vi "UpdateClibWithNewB.vi"(8 "error in (no error)":errorcluster, 11 "MagSpec_Bella in":refnum<class "MagSpec_Bella.lvclass">) -> (0 "error out":errorcluster, 3 "MagSpec_Bella out":refnum<class "MagSpec_Bella.lvclass">)   [LabVIEW 2013, in "MagSpec_Bella.lvclass"]
uses:
  MagSpec_Bella.lvclass
  MagSpec_Bella.lvclass/MagSpec_Bella.ctl
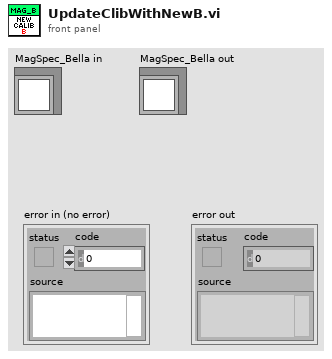
[diagram p1: front panel]
types:
  T1 = typedef "Calibration_Pixel_based.ctl" = cluster{"y1(pixel)":dbl[], "y2(pixel)":dbl[], "dp/B [MeV/C/B] (pixel)":dbl[], "energyDependence Input(pixel)":dbl[], "bending angle [deg](pixel)":dbl[], "total path(pixel)":dbl[], "pixel angle (y)(pixel)":dbl[], "energy dependence (pixel)":dbl[], "charge compensation (pixel)":dbl[], "Momentum [MeV/C](pixel)":dbl[], "angular compensation(pixel)":dbl[]}
  T2 = typedef "CameraSettings_File.ctl" = cluster{"FOV [mm]":dbl, "Left edge [mm]":dbl, "ROI Y offset":dbl, "ROI height":dbl, "ROI X offset":dbl, "ROI width":dbl, "Y center pixel":dbl, "Y Start":dbl, "Y End":dbl, "X Start":dbl, "X End":dbl, "rot [deg]":dbl}
  T3 = typedef "2D.ctl" = cluster{"dp":dbl[][], "chargeCompensation":dbl[][], "angle":dbl[][], "Momentum":dbl[][]}
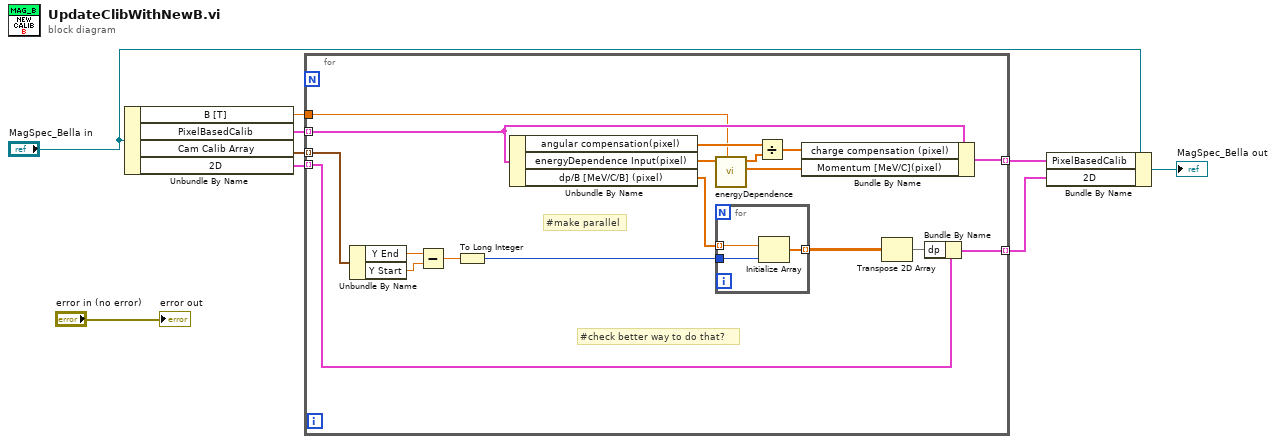
[diagram p0: block diagram]
diagram:
  n1 = Unbundle By Name("MagSpec_Bella in") -> ("B [T]"=w2:dbl, "PixelBasedCalib"=w6:T1[], "Cam Calib Array"=w4:T2[], "2D"=w1:T3[])
  n2 = for {
    tunnel: w6 -> [w24] mode=indexing
    tunnel: [w23] -> w8 mode=indexing
    tunnel: w2 -> [w22]
    tunnel: w1 -> [w18] mode=indexing
    tunnel: [w21] -> w5 mode=indexing
    tunnel: w4 -> [w17] mode=indexing
    # "#check better way to do that?"
    # "#make parallel"
    n3 = Unbundle By Name(w17) -> ("Y End"=w13:dbl, "Y Start"=w12:dbl)
    n4 = Subtract(x=w13, y=w12) -> (x-y=w11:dbl)
    n5 = To Long Integer(number=w11) -> (32bit integer=w16:i32)
    n6 = Unbundle By Name(w24) -> ("angular compensation(pixel)"=w27:dbl[], "energyDependence Input(pixel)"=w26:dbl[], "dp/B [MeV/C/B] (pixel)"=w19:dbl[])
    n7 = call "energyDependence.vi"("B [T]"=w22, "energy Dep in"=w26) -> ("Momentum [MeV/C]"=w25:dbl[], "energy dependence"=w10:dbl[])  [unwired: 8 in]
    n8 = for {
      tunnel: w19 -> [w30] mode=indexing
      tunnel: [w29] -> w20 mode=indexing
      tunnel: w16 -> [w28]
      n9 = Initialize Array(w30, w28) -> (w29:dbl[])
    }
    n10 = Divide(x=w27, y=w10) -> (x/y=w14:dbl[])
    n11 = Bundle By Name(cluster=w24, "charge compensation (pixel)"=w14, "Momentum [MeV/C](pixel)"=w25) -> (w23:T1)
    n12 = Transpose 2D Array(2D array=w20) -> (transposed array=w15:dbl[][])
    n13 = Bundle By Name(cluster=w18, "dp"=w15) -> (w21:T3)
  }
  n14 = Bundle By Name(cluster="MagSpec_Bella in", "PixelBasedCalib"=w8, "2D"=w5) -> (→"MagSpec_Bella out":refnum<class "MagSpec_Bella.lvclass">)
  "error out" <- "error in (no error)"
